vi "EndScan.vi"(8 "error in (no error)":errorcluster caption="entrée d'erreur (pas d'erreur)", 10 "AcqComp":bool, 11 "Experiment en entrée":refnum<class "Experiment.lvclass"> caption="DNL_LabVIEW Object in") -> (0 "error out":errorcluster caption="sortie d'erreur", 2 "PostScanString":string, 3 "Experiment en sortie":refnum<class "Experiment.lvclass"> caption="DNL_LabVIEW Object out")   [LabVIEW 2019, in "Experiment.lvclass"]
uses:
  Experiment.lvclass
  Experiment.lvclass/Experiment.ctl
  DevicesClass/BaseDevice/BaseDevice.lvclass
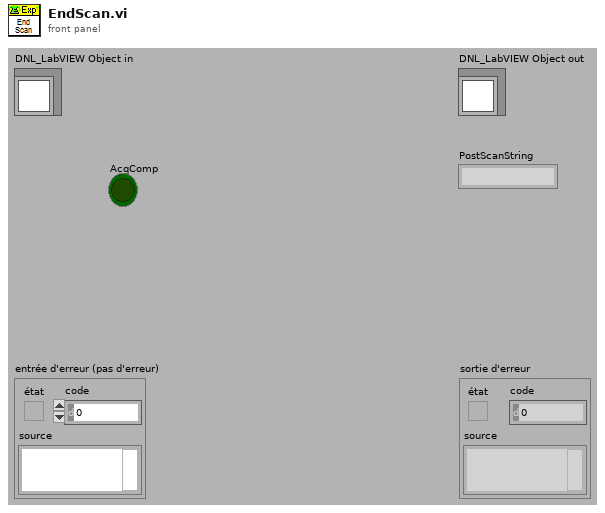
[diagram p1: front panel]
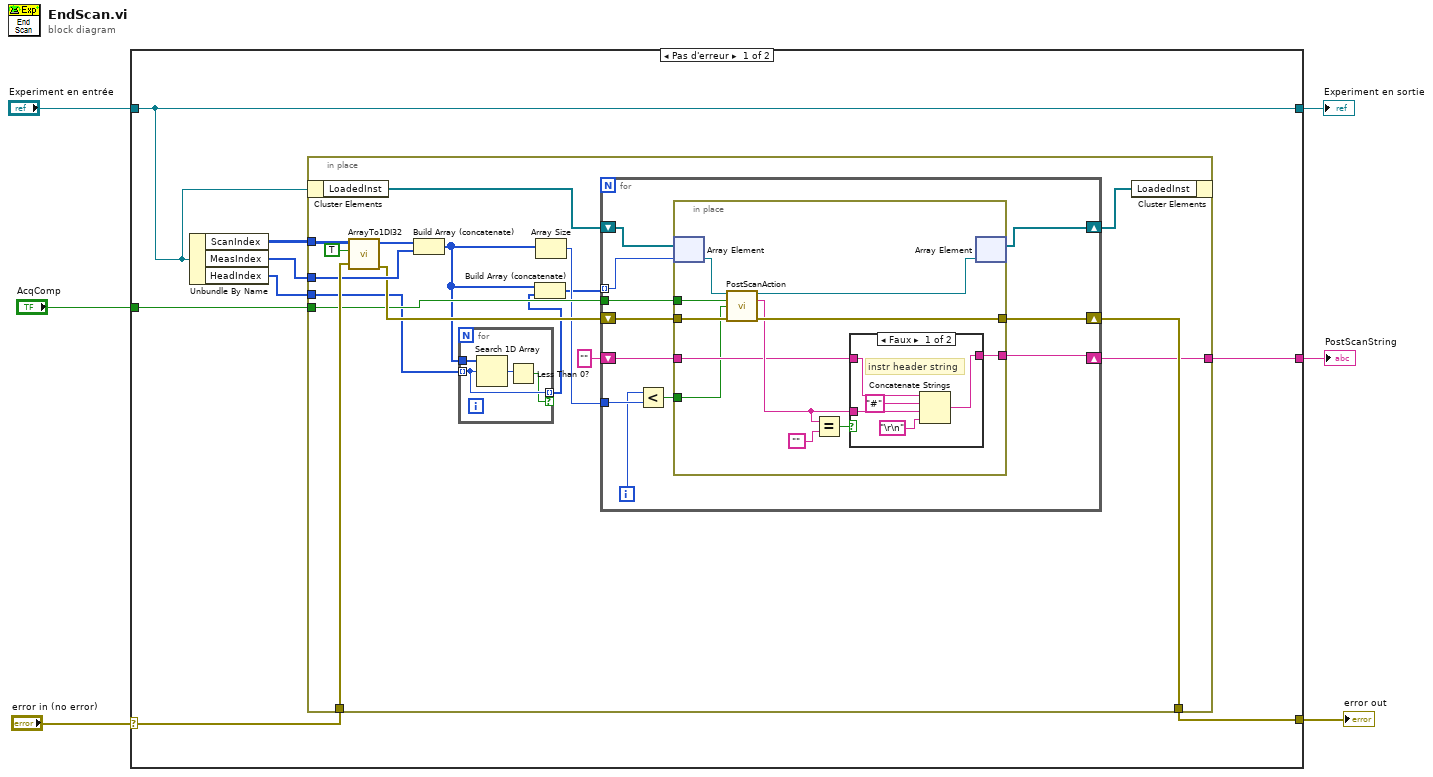
[diagram p0: block diagram]
diagram:
  n1 = case shown="Pas d'erreur" "error in (no error)" {
    selector: "error in (no error)" -> [w13 w65]
    tunnel: [w12 w65] -> w5
    tunnel: [w14 w64] -> w3
    tunnel: "Experiment en entrée" -> [w14 w64]
    tunnel: [w11 _] -> w2
    tunnel: "AcqComp" -> [w10 _]
    frame No Error {
      n2 = Unbundle By Name(w14) -> ("ScanIndex"=w9:i32[][], "MeasIndex"=w8:i32[], "HeadIndex"=w7:i32[])
      n3 = in-place {
        in-place-border: w9 -> [w30]
        in-place-border: w13 -> [w28]
        in-place-border: w8 -> [w27]
        in-place-border: [w23] -> w12
        in-place-border: [w21] -> w11
        in-place-border: w10 -> [w20]
        in-place-border: w7 -> [w17]
        n4 = in-place-cluster #1(w14) -> ("LoadedInst"=w26:refnum<class "BaseDevice.lvclass">[])
        n5 = call <userlib>:"ArrayTo1DI32.vi"("ErrorIn(No Error)"=w28, "DelArrEnd"=TRUE, "tableau"=w30) -> ("sortie d'erreur"=w25:errorcluster, "Array Out"=w29:i32[])  [unwired: 6 in, 1 out]
        n6 = Build Array (concatenate)(w29, w27) -> (w15:i32[])
        n7 = for {
          tunnel: w17 -> [w33] mode=indexing
          tunnel: w15 -> [w35]
          tunnel: [w33] -> w16 mode=indexing if=w32
          n8 = Search 1D Array(1D array=w35, element=w33) -> (index of element=w34:i32)  [unwired: 1 in]
          n9 = Less Than 0?(x=w34) -> (x < 0?=w32:bool)
        }
        n10 = Build Array (concatenate)(w15, w16) -> (w18:i32[])
        n11 = Array Size(array=w15) -> (size(s)=w19:i32)
        n12 = for {
          tunnel: w18 -> [w45] mode=indexing
          shift-right: [w42] -> w24
          shift-left: w26 -> [w46]
          shift-right: [w43] -> w23
          shift-left: w25 -> [w44]
          shift-right: [w41] -> w21
          shift-left: "" -> [w40]
          tunnel: w20 -> [w39]
          tunnel: w19 -> [w37]
          i -> [w36]
          n13 = Less?(x=w36, y=w37) -> (x < y?=w38:bool)
          n14 = in-place {
            in-place-border: w44 -> [w56]
            in-place-border: [w55] -> w43
            in-place-border: [w50] -> w41
            in-place-border: w40 -> [w49]
            in-place-border: w39 -> [w48]
            in-place-border: w38 -> [w47]
            n15 = in-place-array #2(w46, w45) -> (w57:refnum<class "BaseDevice.lvclass">)
            n16 = call-dynamic "PostScanAction.vi"("Device en entrée"=w57, "AcqComp"=w48, "ScanDev"=w47, "error in (no error)"=w56) -> ("Device en sortie"=w54:refnum<class "BaseDevice.lvclass">, "PostScanString"=w51:string, "error out"=w55:errorcluster)  [unwired: 9 in]
            n17 = Equal?(x=w51, y="") -> (x = y?=w53:bool)
            n18 = case shown="Faux" w53 {
              tunnel: [w61 w63] -> w50
              tunnel: w51 -> [w59 _]
              tunnel: w49 -> [w60 w63]
              frame False {
                # "instr header string"
                n19 = Concatenate Strings(w60, "#" ("chaîne"), w59, "\r\n") -> (w61:string)
              }
              frame True {
              }
            }
            n20 = in-place-array #2(w54) -> (w42:refnum<class "BaseDevice.lvclass">[])  [unwired: 1 out]
          }
        }
        n21 = in-place-cluster #1("LoadedInst"=w24) -> ()  [unwired: 1 out]
      }
    }
    frame Error {
    }
  }
  "error out" <- w5
  "Experiment en sortie" <- w3
  "PostScanString" <- w2
